vi "ble_scan_devices.vi"() -> ()   [LabVIEW 2013]
uses:
  type_def/connection_status_bundle.ctl
  type_def/address_type.ctl
panel:
  out "Connected":bool
  out "Device Name":string
  in  "Address Type":T1=1 items=["Public", "Random"]
  out "Handle table":string[][](array[string])
  out "Connection Status":T2={"MAC Address"="", "cnx handle"=0, "cnx flags"=0, "Address Type"=125, "Connection Interval (ms)"=125, "Timeout(ms)"=125, "Latency"=0, "bonding handle"=0} {"Address Type" items=["Public", "Random"]}
  out "Scanning":bool
  in  "Continue":bool
  in  "MAC Address":string
  in  "COM Bluegiga in":refnum<visa-resource-name>="COM13"
  out "Devices":string[][](array[string])
  out "BLED112 Dongle Info":string
  # "This VI an example of scanning for BLE devices using the \nBLED112 Bluetooth Smart Dongle by Bluegiga\nhttps://www.bluegiga.com/en-US/products/bled112-bluetooth-smart-dongle/\n\nand\nBLE (Bluetooth Low Energy) toolkit for LabVIEW\nww.\n\nInstructions:\nBefore running the VI\n1. Select the COM port for the BLED112 USB receiver\n(You can verify this in the Device Manager)\n\n2. Run the VI\n\n3. The VI will reset the dongle and scan for available BLE devices\n \n4. Introduce the MAC Address and Address Type of the device you want to connect and click in the CONTINUE button to connect with it\n\n5. The VI will read the Characteristic 0x2A00 of the Service 0x1800 which contains \nthe Device Name\n\n6. The reversed Device Name will be writen in the Characteristic 0x2A00 of the Service 0x1800\n\nhttps://www.bluetooth.com/specifications/gatt/viewer?attributeXmlFile=org.bluetooth.service.generic_access.xml&u=org.bluetooth.service.generic_access.xml"
  # "SCAN"
  # "RSSI (power)"
  # "Advertising Package Type"
  # "MAC Address"
  # "Address Type"
  # "Friendly name"
  # "DEVICES FOUND"
  # "Introduce the MAC Address and Address Type of the device you want to connect and click in the CONTINUE button"
  # "CONNECT"
  # "READING DEVICE NAME"
  # "Service 0x1800\nCharacteristic 0x2A00\nDevice Name"
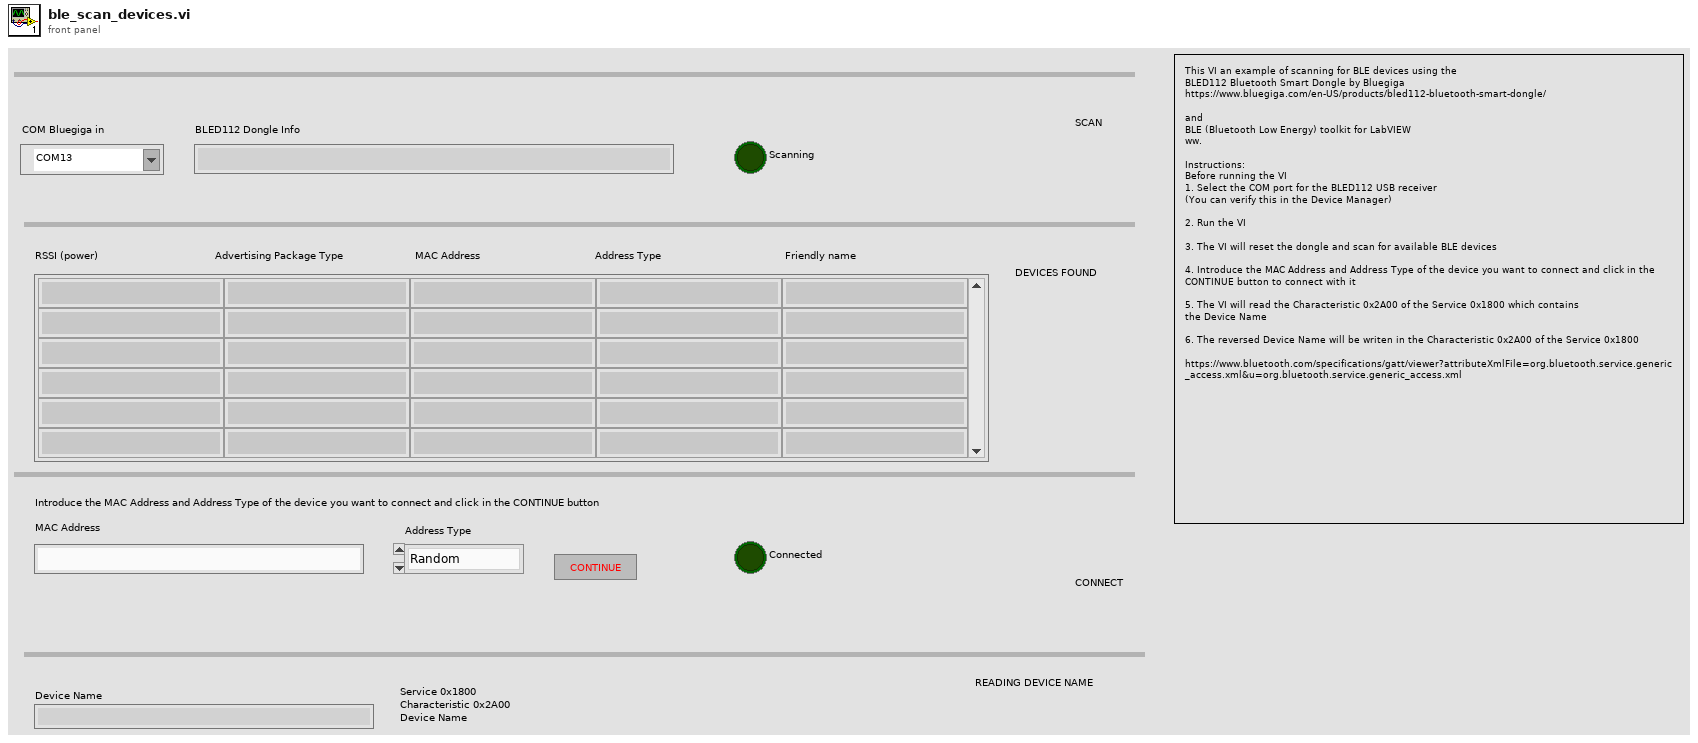
[diagram p1: front panel]
types:
  T1 = typedef "address_type.ctl" = u8
  T2 = typedef "connection_status_bundle.ctl" = cluster{"MAC Address":string, "cnx handle":u8, "cnx flags":u8, "Address Type":T1, "Connection Interval (ms)":u16, "Timeout(ms)":u16, "Latency":u16, "bonding handle":u8}
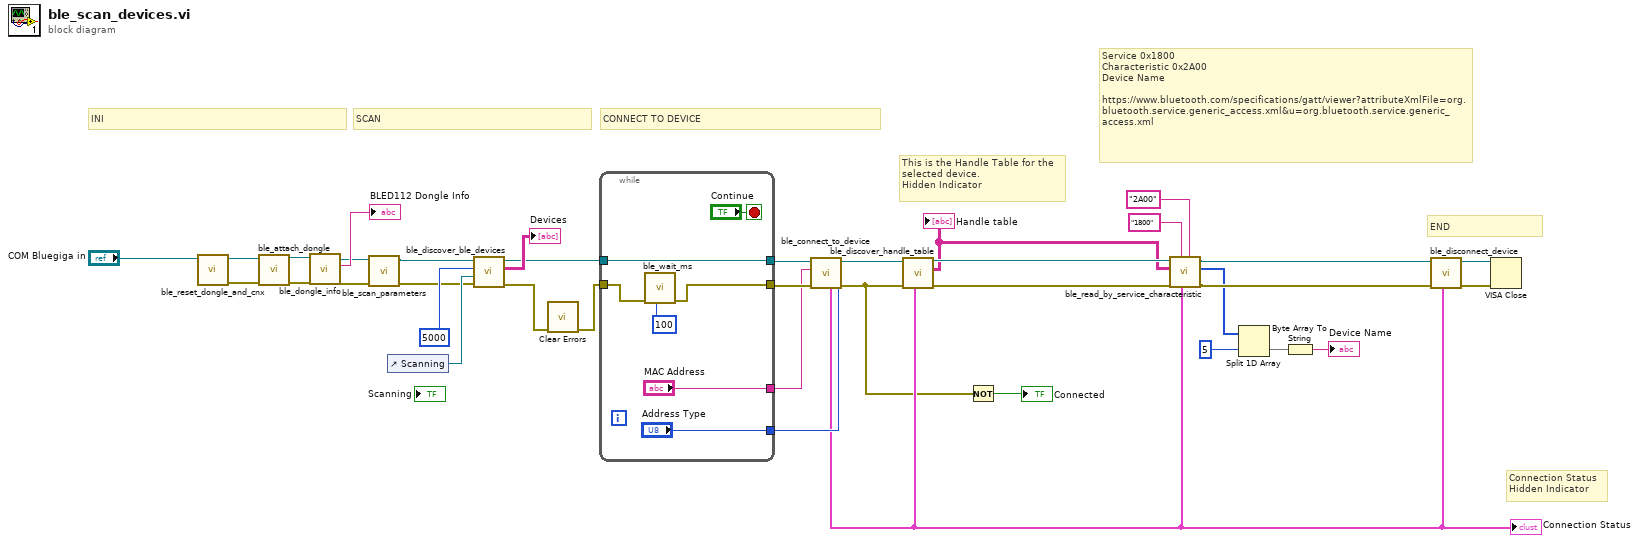
[diagram p0: block diagram]
diagram:
  # "Connection Status\nHidden Indicator"
  # "Service 0x1800\nCharacteristic 0x2A00\nDevice Name\n\nhttps://www.bluetooth.com/specifications/gatt/viewer?attributeXmlFile=org.bluetooth.service.generic_access.xml&u=org.bluetooth.service.generic_access.xml"
  # "This is the Handle Table for the\nselected device. \nHidden Indicator"
  # "CONNECT TO DEVICE"
  # "SCAN"
  # "END"
  # "INI"
  n1 = call "ble_reset_dongle_and_cnx.vi"("COM Bluegiga in"="COM Bluegiga in") -> ("error out"=w21:errorcluster, "COM Bluegiga out"=w19:refnum<visa-resource-name>)  [unwired: 9 in]
  n2 = call "ble_attach_dongle.vi"("error in (no error)"=w21, "COM Bluegiga in"=w19) -> ("error out"=w23:errorcluster, "COM Bluegiga out"=w22:refnum<visa-resource-name>)  [unwired: 8 in]
  n3 = call "ble_dongle_info.vi"("error in (no error)"=w23, "COM Bluegiga in"=w22) -> ("error out"=w29:errorcluster, "info"=→"BLED112 Dongle Info":string, "COM Bluegiga out"=w30:refnum<visa-resource-name>)  [unwired: 7 in]
  n4 = call "ble_scan_parameters.vi"("error in (no error)"=w29, "COM Bluegiga in"=w30) -> ("error out"=w27:errorcluster, "COM Bluegiga out"=w28:refnum<visa-resource-name>)  [unwired: 7 in, 1 out]
  n5 = control-ref of="Scanning"() -> (w33:refnum<vi>)
  n6 = call "ble_discover_ble_devices.vi"("error in (no error)"=w27, "LED ref"=w33, "Scan Duration (10000ms)"=u32 5000, "COM Bluegiga in"=w28) -> ("error out"=w17:errorcluster, "Devices"=→"Devices":string[][], "COM Bluegiga out"=w34:refnum<visa-resource-name>)  [unwired: 5 in]
  n7 = call <vilib>:"Clear Errors.vi"("error in (no error)"=w17) -> ("error out"=w16:errorcluster)  [unwired: 6 in]
  n8 = while {
    tunnel: w16 -> [w43]
    tunnel: [w42] -> w32
    tunnel: w34 -> [w42]
    tunnel: [w41] -> w31
    tunnel: ["MAC Address"] -> w24
    tunnel: ["Address Type"] -> w15
    stop <- "Continue" stop-if-true
    n9 = call "ble_wait_ms.vi"("milliseconds to wait (100)"=u32 100, "error in (no error)"=w43) -> ("error out"=w41:errorcluster)  [unwired: 9 in]
  }
  n10 = call "ble_connect_to_device.vi"("Address Type"=w15, "error in (no error)"=w31, "MAC Address"=w24, "COM Bluegiga in"=w32) -> ("error out"=w1:errorcluster, "COM Bluegiga out"=w18:refnum<visa-resource-name>, "Connection Status"=w7:T2)  [unwired: 5 in]
  "Connection Status" <- w7
  n11 = call "ble_discover_handle_table.vi"("Connection Status"=w7, "error in (no error)"=w1, "COM Bluegiga in"=w18) -> ("error out"=w14:errorcluster, "Handle table"=w12:string[][], "COM Bluegiga out"=w13:refnum<visa-resource-name>)  [unwired: 6 in]
  "Handle table" <- w12
  n12 = Not(x=w1) -> (.not. x?=→"Connected":bool)
  n13 = call "ble_read_by_service_characteristic.vi"("Characteristic UUID"="2A00" ("Service UUID"), "Connection Status"=w7, "Service UUID"="1800", "error in (no error)"=w14, "Handle table"=w12, "COM Bluegiga in"=w13) -> ("error out"=w9:errorcluster, "payload"=w4:u8[], "COM Bluegiga out"=w8:refnum<visa-resource-name>)  [unwired: 2 in, 1 out]
  n14 = Split 1D Array(array=w4, index=5) -> (second subarray=w3:u8[])  [unwired: 1 out]
  n15 = Byte Array To String(unsigned byte array=w3) -> (string=→"Device Name":string)
  n16 = call "ble_disconnect_device.vi"("Connection Status"=w7, "error in (no error)"=w9, "COM Bluegiga in"=w8) -> ("error out"=w25:errorcluster, "COM Bluegiga out"=w26:refnum<visa-resource-name>)  [unwired: 7 in]
  n17 = VISA Close(VISA resource name=w26, error in (no error)=w25) -> ()  [unwired: 1 out]
